vi "Merge Channel Name.vi"(10 "Child":string, 11 "Parent":string) -> (3 "Channel Name":string)   [LabVIEW 2021, in "CIFCoreCommon.lvlib"]
doc: "Channels on the system are a combination of the plugin name followed by a \".\" followed by the channel name. Some channels also contain heirachy with a \".\" seperator. This will merge the parent (typically plugin name) and the child (typically channel name)."
uses:
  CIFCoreCommon.lvlib
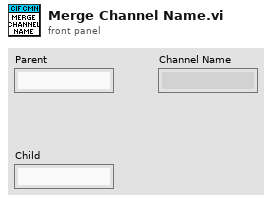
[diagram p1: front panel]
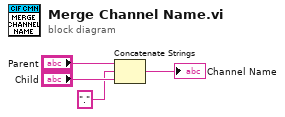
[diagram p0: block diagram]
diagram:
  n1 = Concatenate Strings("Parent", "." ("string"), "Child") -> (→"Channel Name":string)
